vi "Read model.vi"(11 "Context in":refnum<class "Context.lvclass">) -> (2 "Model.lvclass":refnum<class "Model.lvclass">, 3 "Context out":refnum<class "Context.lvclass">)   [LabVIEW 2013, in "Context.lvclass"]
uses:
  Context.lvclass
  Model/Model/Model.lvclass
  Context.lvclass/Context.ctl
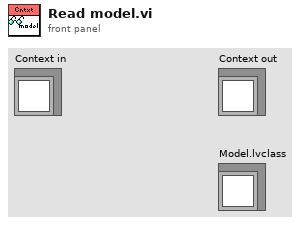
[diagram p1: front panel]
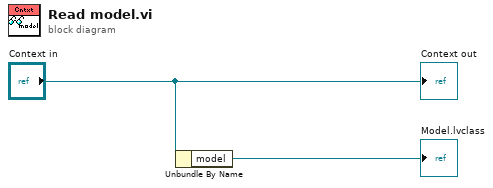
[diagram p0: block diagram]
diagram:
  n1 = Unbundle By Name("Context in") -> ("model"=→"Model.lvclass":refnum<class "Model.lvclass">)
  "Context out" <- "Context in"
